vi "encodeArray.vi"(8 "error in (no error)":errorcluster, 10 "Variant":variant) -> (0 "error out":errorcluster, 2 "Array":u8[](array[numeric]) format="%.0x")   [LabVIEW 2016, in "MsgPack.lvlib"]
uses:
  MsgPack.lvlib
  <vilib>/Utility/error.llb/Error Cluster From Error Code.vi
  <vilib>/ErrorRing/Error Ring.xnode
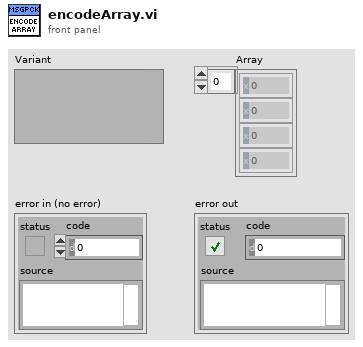
[diagram p1: front panel]
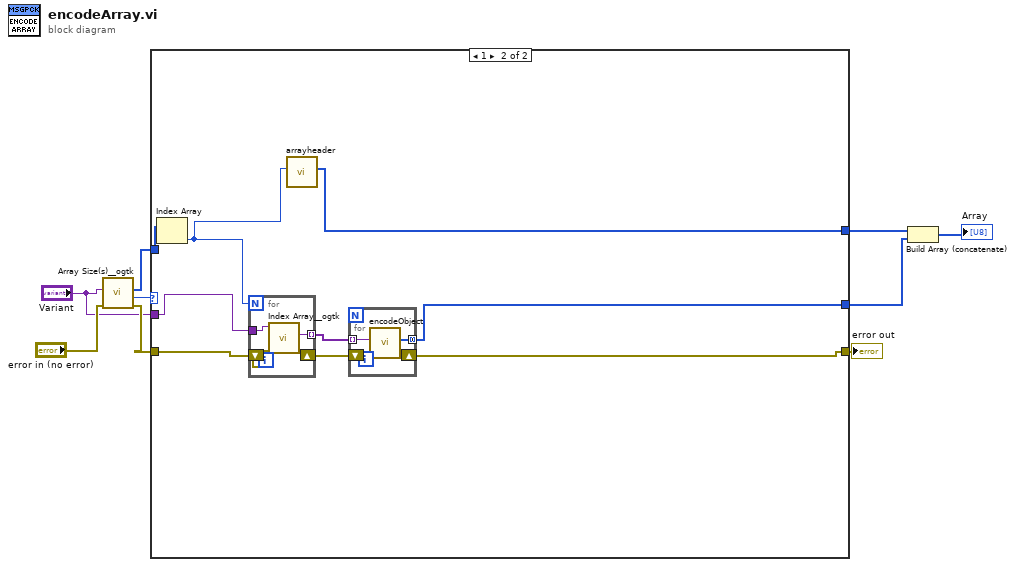
[diagram p0: block diagram]
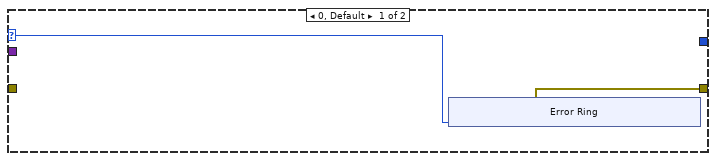
[diagram p2: hidden frame]
diagram:
  n1 = call <userlib>:"Array Size(s)__ogtk.vi"("error in (no error)"="error in (no error)", "Array"="Variant") -> ("error out"=w7:errorcluster, "N dims"=w5:u32, "Size(s)"=w6:u32[])  [unwired: 7 in]
  n2 = case shown="1" w5 {
    selector: w5 -> [w10 _]
    tunnel: [_ w19] -> w2
    tunnel: w7 -> [_ w27]
    tunnel: w6 -> [_ w26]
    tunnel: [w11 w24] -> w4
    tunnel: "Variant" -> [_ w25]
    tunnel: [_ w23] -> w1
    frame 0, Default {
      n3 = xnode "Error Ring"("parameter 0"=w10) -> ("error out"=w11:errorcluster)
    }
    frame 1 {
      n4 = Index Array(array=w26) -> (element=w20:u32)  [unwired: 1 in]
      n5 = for {
        N: w20 -> [_]
        tunnel: w25 -> [w34]
        tunnel: [w33] -> w21 mode=indexing
        shift-right: [w32] -> w22
        shift-left: w27 -> [w35]
        n6 = call <userlib>:"Index Array__ogtk.vi"("error in (no error)"=w35, "MultiD Array"=w34) -> ("error out"=w32:errorcluster, "Array Element"=w33:variant)  [unwired: 8 in]
      }
      n7 = call "arrayheader.vi"("Numeric"=w20) -> ("header"=w19:u8[])  [unwired: 10 in]
      n8 = for {
        tunnel: w21 -> [w29] mode=indexing
        shift-right: [w31] -> w24
        shift-left: w22 -> [w30]
        tunnel: [w28] -> w23 mode=concatenating
        n9 = call "encodeObject.vi"("error in (no error)"=w30, "Variant"=w29) -> ("error out"=w31:errorcluster, "Array"=w28:u8[])  [unwired: 8 in]
      }
    }
  }
  "error out" <- w4
  n10 = Build Array (concatenate)(w2, w1) -> (→"Array":u8[])
